vi "Update Item.vi"(8 "error in (no error)":errorcluster, 9 "New Item":refnum<class "Data Item.lvclass">, 11 "Tree Manager in":refnum<class "Tree Manager.lvclass">) -> (0 "error out":errorcluster, 3 "Tree Manager out":refnum<class "Tree Manager.lvclass">)   [LabVIEW 2026, in "VILab.lvlib" / "Tree Manager.lvclass"]
uses:
  Tree Manager.lvclass
  Tree Manager.lvclass/Tree Manager.ctl
  Data Item/Data Item.lvclass
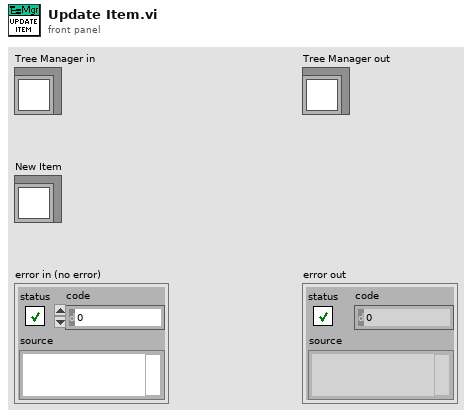
[diagram p1: front panel]
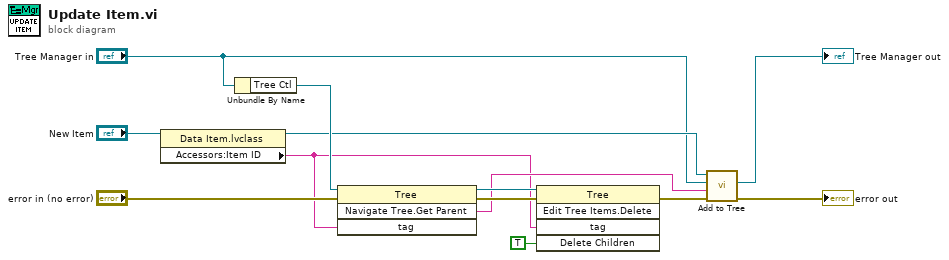
[diagram p0: block diagram]
diagram:
  n1 = property class="Data Item.lvclass"(reference="New Item") -> (reference out=w2:refnum<class "Data Item.lvclass">, "Accessors:Item ID"=w3:string)  [unwired: 1 in, 1 out]
  n2 = Unbundle By Name("Tree Manager in") -> ("Tree Ctl"=w7:refnum<vi>)
  n3 = invoke class="Tree" method="Navigate Tree.Get Parent"(reference=w7, error in="error in (no error)", "tag"=w3) -> (reference out=w6:refnum<vi>, error out=w5:errorcluster, "Navigate Tree:Get Parent"=w4:string)  [unwired: 1 in, 1 out]
  n4 = invoke on="Delete" class="Tree" method="Edit Tree Items.Delete"(reference=w6, error in=w5, "tag"=w3, "Delete Children"=TRUE ("Delete Children?")) -> (error out=w8:errorcluster)  [unwired: 1 in, 4 out]
  n5 = call-dynamic "Add to Tree.vi"("error in (no error)"=w8, "Parent Tag"=w4, "Tree Manager in"="Tree Manager in", "Data Item in"=w2) -> ("error out"=→"error out":errorcluster, "Tree Manager out"=→"Tree Manager out":refnum<class "Tree Manager.lvclass">)  [unwired: 5 in, 1 out]
